vi "Main-Page.vi"() -> ()   [LabVIEW 2015]
uses:
  2.Queue/Control_Main_Queue Action.ctl
  <vilib>/Utility/miscctls.llb/LVPointTypeDef.ctl
  2.0_Function/Function_VISA/Control/Control_Axis Number.ctl
panel:
  out "data":T1(ring)
  in  "使用者帳戶":path=path "D:/全域高斯機 參數/use history"
  in  "參數設定":path=path "D:/全域高斯機 參數/use history"
  out "狀態：":string="可使用"
  out "群組：":string="開發人員"
  in  "原點資訊":path=path "D:/全域高斯機 參數/Original"
  in  "匯入硬體參數":path=path "D:/全域高斯機 參數/use history"
  in  "儲存檔案路徑":path=path "D:/全域高斯機Data"
  in  "匯入圖檔(Setting)":path=path "D:/全域高斯機資料/TAHOE3.png"
  out "狀態：":T2
  in  "離開程式":bool
  out "群組：":T3
  out "帳號：":string="admin"
  out "Queue Action":T4=enum."    10.2 系統-等待"
  in  "關於本系統":bool
  in  "資料管理":bool
  in  "登出/離開":bool
  in  "系統管理選單":bool
  in  "開始":bool
  in  "每日檢測":bool
  # "C:\\Users\\jyun.huang.MINAIK\\Desktop\\四穴雷切\\參數設定\\Data\\參數設定"
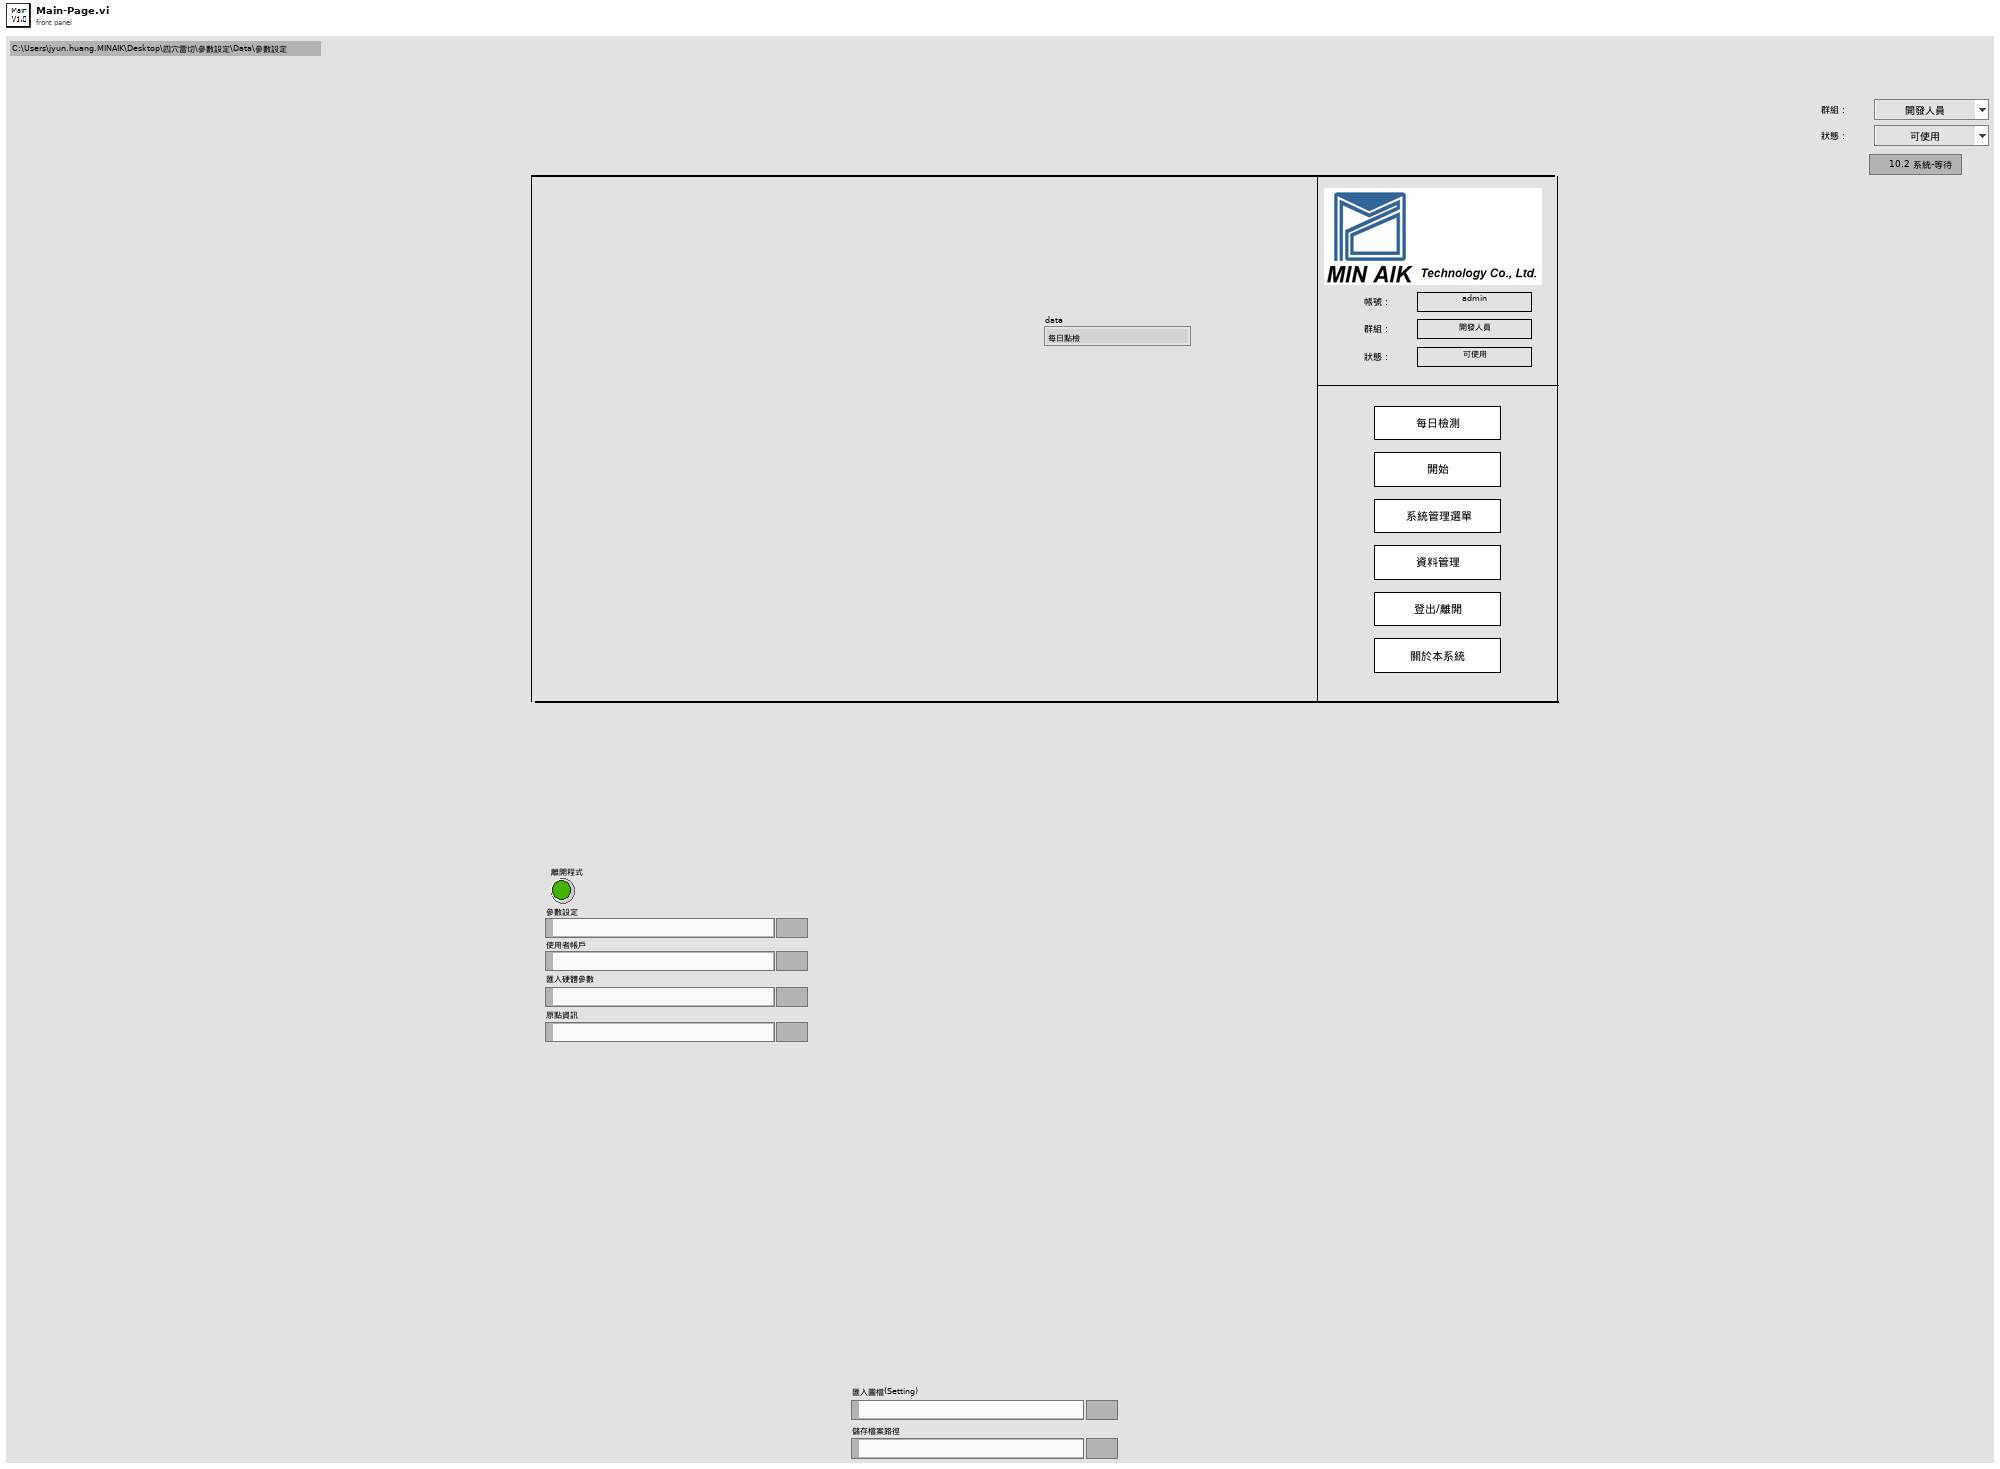
[diagram p1: front panel]
types:
  T1 = enum16{"每日點檢", "開始", "系統管理選單", "資料管理", "登出/離開", "關於本系統"}
  T2 = typedef "Control_User Accounts_Status.ctl" = enum16{"可使用", "不可使用"}
  T3 = typedef "Control_User account_Permissions.ctl" = enum16{"開發人員", "管理者", "工程師", "作業員"}
  T4 = typedef "Control_Main_Queue Action.ctl" = enum16{"動作-使用者登入", "動作-系統初始化", "動作-開始", "動作-系統管理選單", "動作-資料管理", "動作-登出/離開", "動作-關於本系統", "1.0 帳號管理", "    1.1 登入", "    1.2 確認狀態", "    1.3 更新介面", "    1.4 帳號管理", "    1.5 登出", "2.0 每日點檢", "10.0 系統", "    10.1 系統-關機", "    10.2 系統-等待", "    10.3 系統-回到作業系統"}
  T5 = cluster{string, "按鈕":enum16{"每日點檢", "開始", "系統管理選單", "資料管理", "登出/離開", "關於本系統"}}
  T6 = cluster{string, "系統":enum16{"關機", "等待", "回到作業系統"}}
  T7 = cluster{string, "帳號管理":enum16{"登入", "確認狀態", "更新介面", "帳號管理", "登出"}}
  T8 = typedef "LVPointTypeDef.ctl" = cluster{"Horizontal":i16, "Vertical":i16}
  T9 = typedef "Control_Original.ctl" = cluster{"R":dbl, "Y":dbl, "Z":dbl, "Angle":dbl}
  T10 = typedef "Control_軸參數.ctl" = cluster{"Name":string, "VISA In":refnum<visa-resource-name>, "R":dbl, "Y":dbl, "Z":dbl, "θ":dbl, "最大值":dbl, "最小值":dbl, "VISA Data":cluster{"Baud rate":u32, "Data bits":u16, "Parity":enum16{"None", "Odd", "Even", "Mark", "Space"}, "Stop bits":u16, "Flow control":u16}, "Paremeter":T11, "DAQ Paremeter":cluster{"Task In":refnum<k21>, "Physical Channels":tag, "Max Value":dbl, "Min Value":dbl, "Rate":dbl}}
  T11 = typedef "Control_手動測試_軸參數.ctl" = cluster{"Scan speed":T12, "Power":u16, "Angle":dbl, "X":i32, "X":i32, "Xc":i32}
  T12 = typedef "Control_Axis Number.ctl" = u16
  T13 = typedef "Control_Main_All Data.ctl" = enum16{"Initialize", "Set Data", "Get Data"}
  T14 = typedef "Use History.ctl" = enum16{"Initialize", "Set Data", "Get Data", "Idle"}
  T15 = typedef "Control_User account_Data.ctl" = cluster{"帳號 :":string, "權限等級：":T3, "建立時間：":string, "修改時間：":string, "到期時間：":string, "狀態：":T2, "期限：":T16, "密碼：":string}
  T16 = typedef "Control_User account_Date.ctl" = enum16{"零天", "一天", "七天", "一個月", "一年", "三年"}
  T17 = typedef "Action_Data.ctl" = enum16{"Initialize", "Get Data", "Set Data", "Delete Data", "Idle"}
  T18 = cluster{cluster{"掃描速度":i32, "功率":i32, "切割刀數":dbl, "左/右":string}, cluster{"掃描速度2":i32, "功率2":i32, "切割刀數2":dbl, "左/右":string}, cluster{"掃描速度3":i32, "功率3":i32, "切割刀數3":dbl, "左/右":string}, cluster{"掃描速度4":i32, "功率4":i32, "切割刀數4":dbl, "左/右":string}, cluster{"掃描速度5":i32, "功率5":i32, "切割刀數5":dbl, "左/右":string}}
  T19 = enum16{"All Enable", "All Disable", "Port Enable", "Port Disable"}
  T20 = typedef "Control_Bounce Window_Main_System Configuration.ctl" = enum16{"帳號管理", "手動操作", "機器參數設定", "離開", "等待"}
  T21 = typedef "Control_Bounce Window_Main_Data Management.ctl" = enum16{"量測參數設定", "操作履歷", "數據回顧", "離開", "等待"}
  T22 = typedef "Control_Bounce Window_Main_Log On-Exit.ctl" = enum16{"回到作業系統", "關機", "使用者登出", "離開", "等待"}
  T23 = cluster{"掃描速度5":i32, "功率5":i32, "切割刀數5":dbl, "左/右":string}
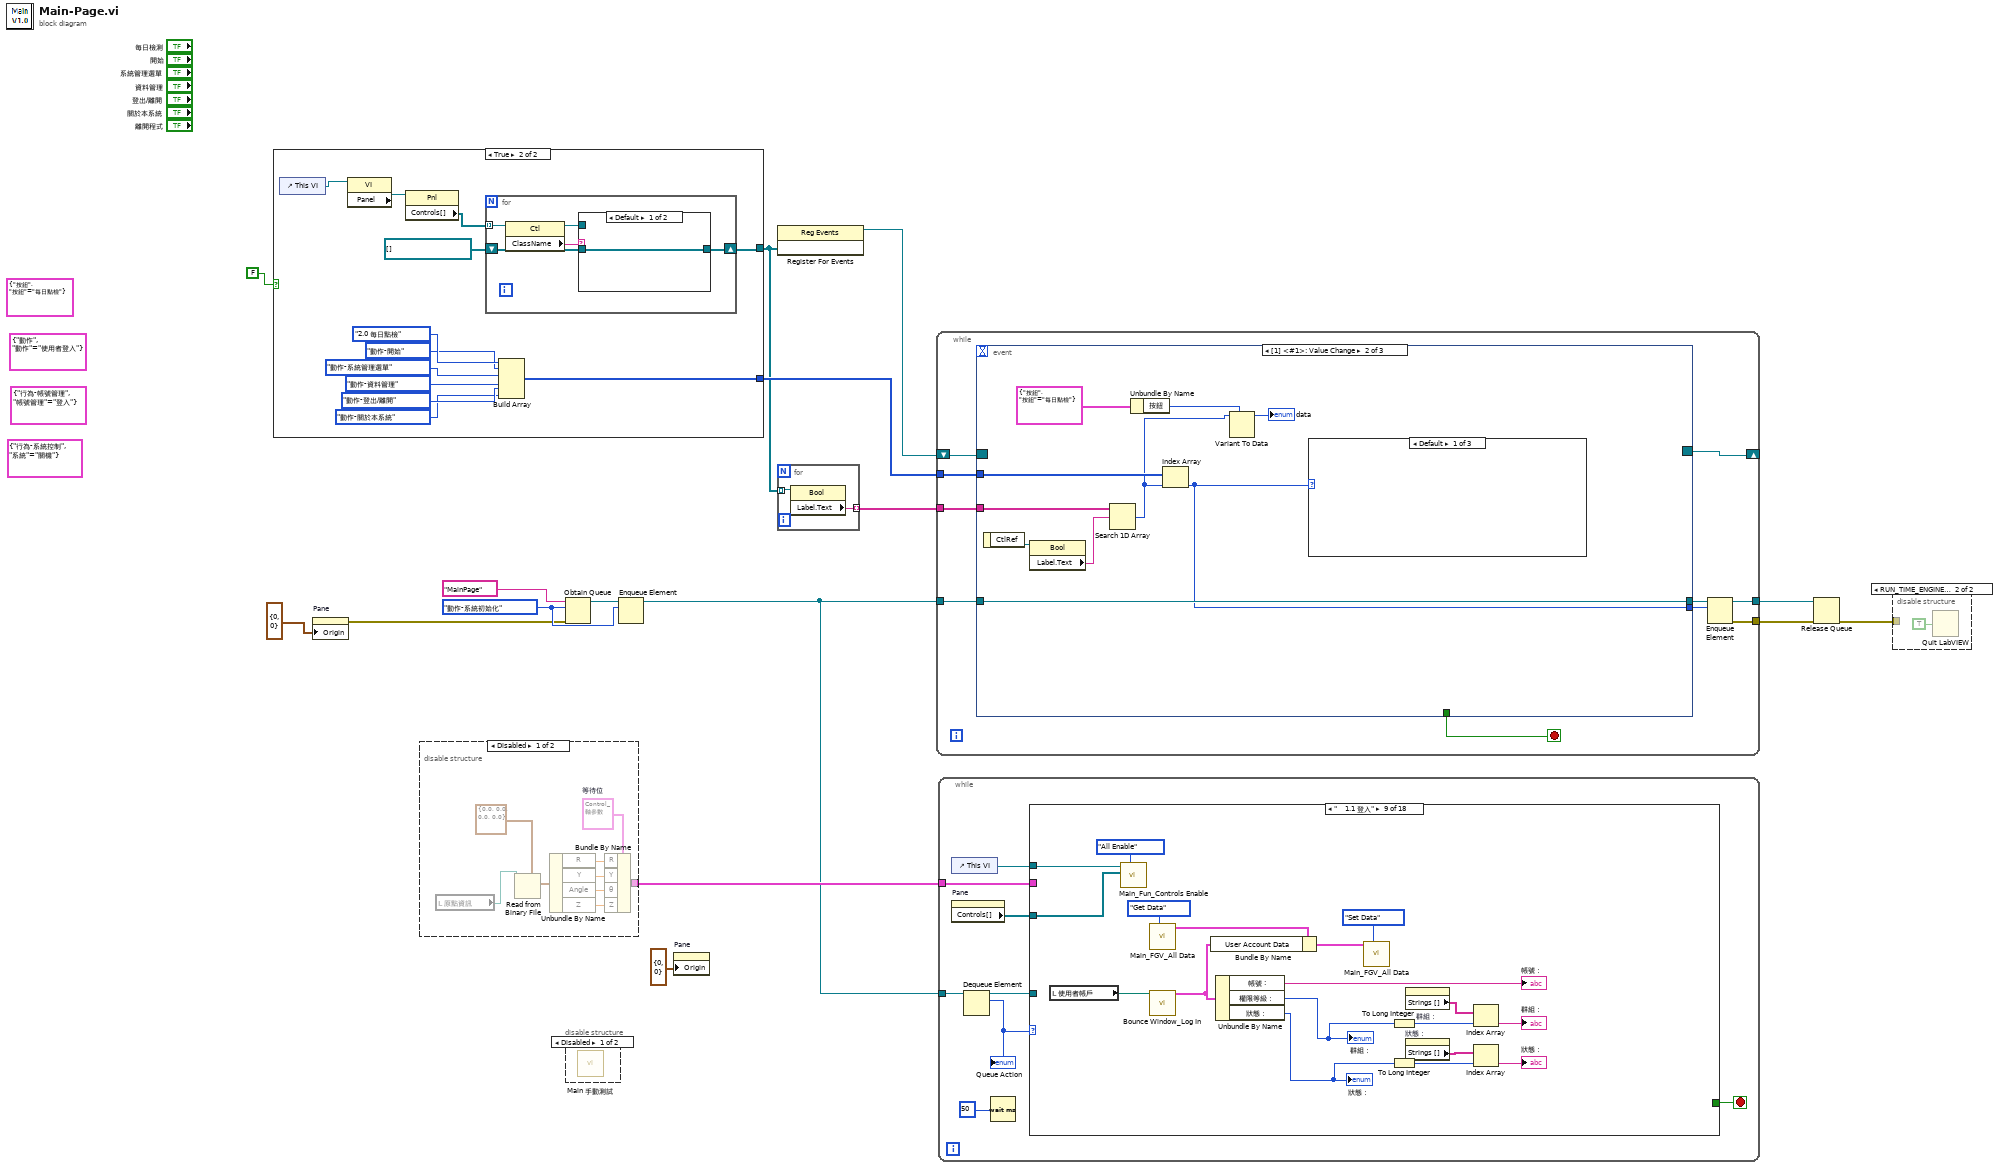
[diagram p0: block diagram]
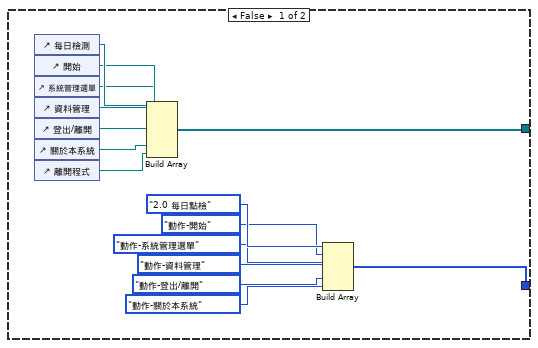
[diagram p2: hidden frame]
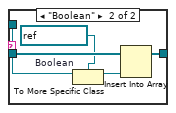
[diagram p3: hidden frame]
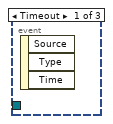
[diagram p4: hidden frame]
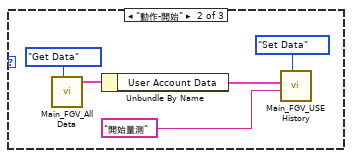
[diagram p5: hidden frame]
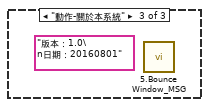
[diagram p6: hidden frame]
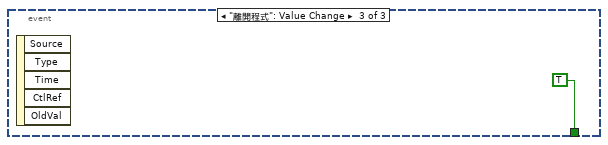
[diagram p7: hidden frame]
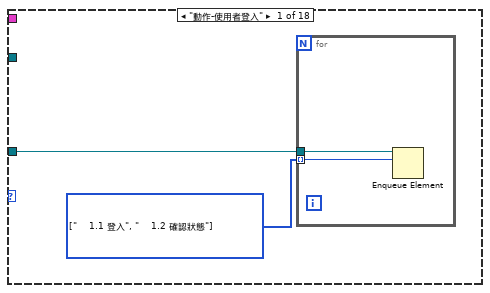
[diagram p11: hidden frame]
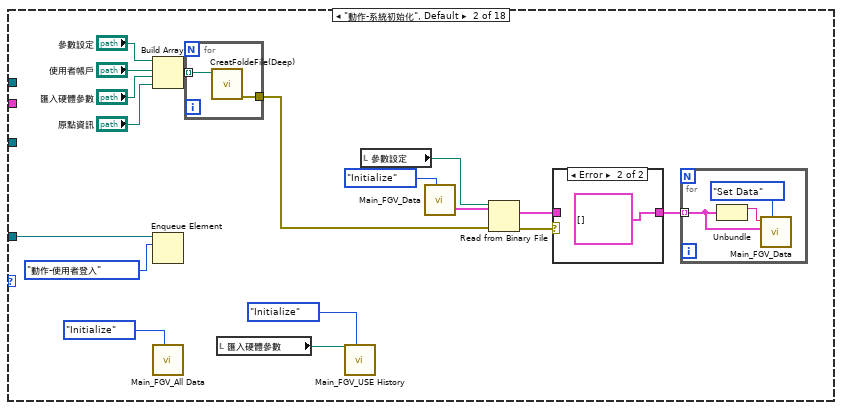
[diagram p12: hidden frame]
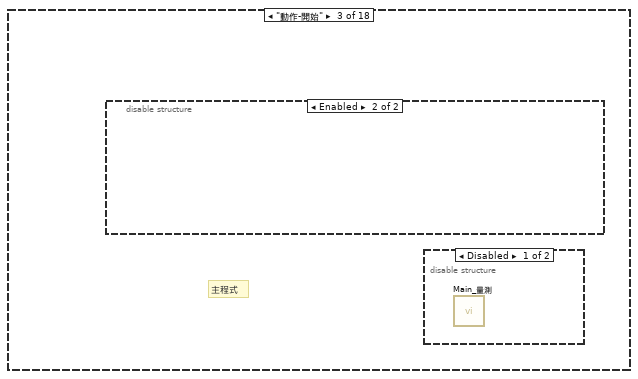
[diagram p14: hidden frame]
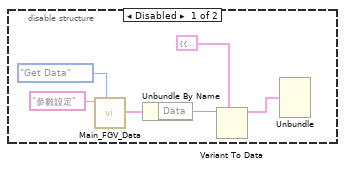
[diagram p16: hidden frame]
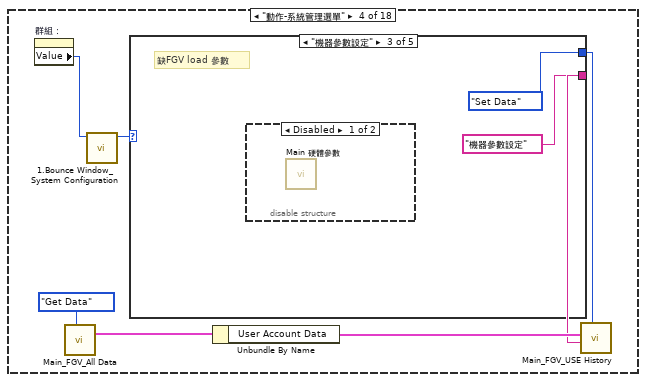
[diagram p17: hidden frame]
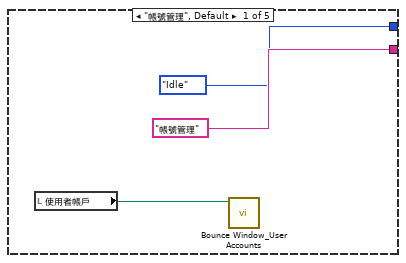
[diagram p18: hidden frame]
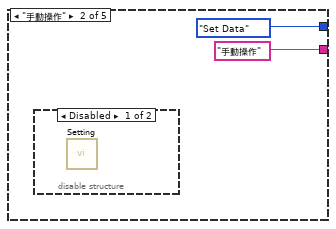
[diagram p19: hidden frame]
diagram:
  (unwired) T5 {"按鈕", "按鈕"=enum."每日點檢"} ("output cluster")
  (unwired) T6 {"行為-系統控制", "系統"=enum."關機"} ("output cluster")
  (unwired) T7 {"行為-帳號管理", "帳號管理"=enum."登入"} ("output cluster")
  (unwired) cluster{string, "動作":enum16{"使用者登入", "系統初始化"}} {"動作", "動作"=enum."使用者登入"} ("output cluster")
  w11 = Control_Main_Queue_Action."動作-系統初始化" ("Queue Action")
  n1 = case shown="True" FALSE {
    tunnel: [w17 w39] -> w3
    tunnel: [w18 w32] -> w6
    frame False {
      n2 = control-ref of="每日檢測"() -> (w31:refnum<vi>)
      n3 = control-ref of="開始"() -> (w30:refnum<vi>)
      n4 = control-ref of="系統管理選單"() -> (w29:refnum<vi>)
      n5 = control-ref of="資料管理"() -> (w28:refnum<vi>)
      n6 = control-ref of="登出/離開"() -> (w27:refnum<vi>)
      n7 = control-ref of="關於本系統"() -> (w26:refnum<vi>)
      n8 = control-ref of="離開程式"() -> (w25:refnum<vi>)
      n9 = Build Array(w31, w30, w29, w28, w27, w26, w25) -> (w17:refnum<vi>[])
      n10 = Build Array(Control_Main_Queue_Action."2.0 每日點檢" ("Queue Action"), Control_Main_Queue_Action."動作-開始" ("Queue Action"), Control_Main_Queue_Action."動作-系統管理選單" ("Queue Action"), Control_Main_Queue_Action."動作-資料管理" ("Queue Action"), Control_Main_Queue_Action."動作-登出/離開" ("Queue Action"), Control_Main_Queue_Action."動作-關於本系統" ("Queue Action")) -> (w18:T4[])
    }
    frame True {
      n11 = control-ref of="This VI"() -> (w43:refnum<vi>)
      n12 = property class="VI"(reference=w43) -> ("Panel"=w42:refnum<vi>)  [unwired: 1 in, 2 out]
      n13 = property class="Pnl"(reference=w42) -> ("Controls[]"=w41:refnum<vi>[])  [unwired: 1 in, 2 out]
      n14 = for {
        tunnel: w41 -> [w46] mode=indexing
        shift-right: [w45] -> w39
        shift-left: refnum<vi>[] [] -> [w47]
        n15 = property class="Ctl"(reference=w46) -> ("ClassName"=w44:string)  [unwired: 1 in, 2 out]
        n16 = case shown="Default" w44 {
          tunnel: w47 -> [w48 w53]
          tunnel: w46 -> [_ w52]
          tunnel: [w48 w50] -> w45
          frame Default {
          }
          frame "Boolean" {
            w51 = refnum<vi> refnum  # Boolean
            n17 = To More Specific Class(target class=w51, reference=w52) -> (specific class reference=w49:refnum<vi>)  [unwired: 1 in, 1 out]
            n18 = Insert Into Array(array=w53, new element=w49) -> (w50:refnum<vi>[])  [unwired: 1 in]
          }
        }
      }
      n19 = Build Array(Control_Main_Queue_Action."2.0 每日點檢" ("Queue Action"), Control_Main_Queue_Action."動作-開始" ("Queue Action"), Control_Main_Queue_Action."動作-系統管理選單" ("Queue Action"), Control_Main_Queue_Action."動作-資料管理" ("Queue Action"), Control_Main_Queue_Action."動作-登出/離開" ("Queue Action"), Control_Main_Queue_Action."動作-關於本系統" ("Queue Action")) -> (w32:T4[])
    }
  }
  n20 = property on="Pane" class="Pane"("Origin"=T8 {"Horizontal"=0, "Vertical"=0}) -> (error out=w10:errorcluster)  [unwired: 2 in, 1 out]
  n21 = disable-structure shown="Disabled" {
    disable-tunnel: [w55 _] -> w14
    frame Disabled {
      w56 = T10 {"Name"="", "VISA In"="COM2", "R"=40.8, "Y"=12.9, "Z"=0.0, "θ"=87.62, "最大值"=0.0, "最小值"=0.0, "VISA Data"={"Baud rate"=115200, "Data bits"=8, "Parity"=enum."Even", "Stop bits"=10, "Flow control"=0}, "Paremeter"={"Scan speed"=4, "Power"=2, "Angle"=0.0, "X"=9000, "X"=60000, "Xc"=60000}, "DAQ Paremeter"={"Task In"="CalibrationTest", "Physical Channels"="Dev1/ai0", "Max Value"=10.0, "Min Value"=-10.0, "Rate"=1000.0}}  # 等待位
      n22 = local read "原點資訊"() -> (w54:path)
      n23 = Read from Binary File(5:T9 {"R"=0.0, "Y"=0.0, "Z"=0.0, "Angle"=0.0} ("治具原點"), 11:w54) -> (2:w61:T9)  [unwired: 4 in, 3 out]
      n24 = Unbundle By Name(w61) -> ("R"=w60:dbl, "Y"=w59:dbl, "Angle"=w58:dbl, "Z"=w57:dbl)
      n25 = Bundle By Name(cluster=w56, "R"=w60, "Y"=w59, "θ"=w58, "Z"=w57) -> (w55:T10)
    }
    frame Enabled {
    }
  }
  n26 = Obtain Queue(name (unnamed)="MainPage", element data type=w11, error in (no error)=w10) -> (queue out=w12:refnum<queue>)  [unwired: 2 in, 2 out]
  n27 = disable-structure shown="Disabled" {
    frame Disabled {
      n28 = call "Main 手動測試.vi"() -> ()  [unwired: 12 in]
    }
    frame Enabled {
    }
  }
  n29 = Enqueue Element(queue=w12, element=w11) -> (queue out=w7:refnum<queue>)  [unwired: 2 in, 2 out]
  n30 = property on="Pane" class="Pane"("Origin"=T8 {"Horizontal"=0, "Vertical"=0}) -> ()  [unwired: 2 in, 2 out]
  n31 = register-events(w3) -> (reference out=w9:refnum<event-registration>)  [unwired: 2 in, 1 out]
  n32 = for {
    tunnel: w3 -> [w64] mode=indexing
    tunnel: [w63] -> w2 mode=indexing
    n33 = property class="Bool"(reference=w64) -> ("Label.Text"=w63:string)  [unwired: 1 in, 2 out]
  }
  n34 = while {
    shift-right: [w73] -> _
    shift-left: w9 -> [w74]
    tunnel: w2 -> [w72]
    tunnel: w7 -> [w70]
    tunnel: w6 -> [w68]
    tunnel: [w67] -> w5
    tunnel: [w66] -> w4
    stop <- w65 stop-if-true
    n35 = event shown="[1] <#1>: Value Change" {
      selector: w74 -> [_ _ _]
      dyn-events: [_ _ _] -> w73
      timeout: _ -> [_ _ _]
      tunnel: w72 -> [_ w84 _]
      tunnel: [_ w82 _] -> w71
      tunnel: w70 -> [_ w82 _]
      tunnel: [_ w76 _] -> w69
      tunnel: w68 -> [_ w81 _]
      tunnel: [_ _ TRUE] -> w65
      event Timeout {
        n36 = event-data() -> ()  [unwired: 1 in, 3 out]
      }
      event Value Change {
        n37 = event-data() -> ("CtlRef"=w80:refnum<vi>)  [unwired: 1 in]
        n38 = property class="Bool"(reference=w80) -> ("Label.Text"=w83:string)  [unwired: 1 in, 2 out]
        n39 = Search 1D Array(1D array=w84, element=w83) -> (index of element=w75:i32)  [unwired: 1 in]
        n40 = Unbundle By Name(T5 {"按鈕", "按鈕"=enum."每日點檢"} ("output cluster")) -> ("按鈕"=w78:T1)
        n41 = Index Array(array=w81, index=w75) -> (element=w76:T4)
        n42 = Variant To Data(type=w78, Variant=w75) -> (data=→"data":T1)  [unwired: 1 in, 1 out]
        n43 = case shown="Default" w76 {
          frame Default {
          }
          frame "動作-開始" {
            n44 = call "Main_FGV_All Data.vi"("Data_Action"=Control_Main_All_Data."Get Data") -> ("All Data Out"=w85:cluster{"User Account Data":T15})  [unwired: 9 in, 1 out]
            n45 = Unbundle By Name(w85) -> ("User Account Data"=w88:T15)
            n46 = call "Main_FGV_USE History.vi"("Use Action"=Use_History."Set Data", "Event"="開始量測", "User Account Data"=w88) -> ()  [unwired: 8 in, 1 out]
          }
          frame "動作-關於本系統" {
            (unwired) "版本：1.0\n日期：20160801" ("MSG In")
            n47 = call "5.Bounce Window_MSG.vi"() -> ()  [unwired: 12 in]
          }
        }
      }
      event "離開程式": Value Change {
        n48 = event-data() -> ()  [unwired: 1 in, 5 out]
      }
    }
    n49 = Enqueue Element(queue=w71, element=w69) -> (queue out=w67:refnum<queue>, error out=w66:errorcluster)  [unwired: 2 in, 1 out]
  }
  n50 = while {
    tunnel: w7 -> [w93]
    tunnel: w14 -> [w95]
    stop <- w98 stop-if-true
    n51 = control-ref of="This VI"() -> (w97:refnum<vi>)
    n52 = property on="Pane" class="Pane"() -> ("Controls[]"=w96:refnum<vi>[])  [unwired: 2 in, 2 out]
    n53 = Dequeue Element(queue=w93) -> (queue out=w92:refnum<queue>, element=w91:T4)  [unwired: 2 in, 2 out]
    "Queue Action" <- w91
    n54 = Wait (ms)(milliseconds to wait=u32 50) -> ()  [unwired: 1 out]
    n55 = case shown="\"    1.1 登入\"" w91 {
      tunnel: [_ _ _ _ _ _ _ _ _ _ _ _ _ _ TRUE _ TRUE _] -> w98
      tunnel: w92 -> [w100 w104 _ _ _ w166 _ _ _ w215 _ _ _ _ _ _ _ _]
      tunnel: w97 -> [_ _ _ _ _ _ _ _ w197 w209 _ _ _ _ _ _ _ _]
      tunnel: w96 -> [_ _ _ _ _ _ _ _ w196 w208 _ _ _ _ _ _ _ _]
      tunnel: w95 -> [_ _ _ _ w151 _ _ _ _ _ _ _ _ _ _ _ _ _]
      frame "動作-使用者登入" {
        w99 = T4[] [enum."    1.1 登入", enum."    1.2 確認狀態"] items=["動作-使用者登入", "動作-系統初始化", "動作-開始", "動作-系統管理選單", "動作-資料管理", "動作-登出/離開", "動作-關於本系統", "1.0 帳號管理", "    1.1 登入", "    1.2 確認狀態", "    1.3 更新介面", "    1.4 帳號管理", "    1.5 登出", "2.0 每日點檢", "10.0 系統", "    10.1 系統-關機", "    10.2 系統-等待", "    10.3 系統-回到作業系統"]
        n56 = for {
          tunnel: w100 -> [w102]
          tunnel: w99 -> [w101] mode=indexing
          n57 = Enqueue Element(queue=w102, element=w101) -> ()  [unwired: 2 in, 3 out]
        }
      }
      frame "動作-系統初始化", Default {
        n58 = Build Array("參數設定", "使用者帳戶", "匯入硬體參數", "原點資訊") -> (w119:path[])
        n59 = Enqueue Element(queue=w104, element=Control_Main_Queue_Action."動作-使用者登入" ("Queue Action")) -> ()  [unwired: 2 in, 3 out]
        n60 = call "Main_FGV_All Data.vi"("Data_Action"=Control_Main_All_Data."Initialize") -> ()  [unwired: 9 in, 2 out]
        n61 = for {
          tunnel: w119 -> [w126] mode=indexing
          tunnel: [w125] -> w110
          n62 = call "CreatFoldeFile(Deep).vi"("Path"=w126) -> ("error out"=w125:errorcluster)  [unwired: 8 in, 2 out]
        }
        n63 = local read "匯入硬體參數"() -> (w109:path)
        n64 = call "Main_FGV_USE History.vi"("Use Action"=Use_History."Initialize", "匯入硬體參數"=w109) -> ()  [unwired: 9 in, 1 out]
        n65 = local read "參數設定"() -> (w112:path)
        n66 = call "Main_FGV_Data.vi"("Action_Data"=Action_Data."Initialize") -> ("Data Array out"=w111:cluster{"Data name":string, "Data":variant}[])  [unwired: 9 in, 1 out]
        n67 = Read from Binary File(5:w111, 8:w110, 11:w112) -> (0:w107:errorcluster, 2:w106:cluster{"Data name":string, "Data":variant}[])  [unwired: 3 in, 2 out]
        n68 = case shown="Error" w107 {
          tunnel: w106 -> [w120 _]
          tunnel: [w120 cluster{"Data name":string, "Data":variant}[] [] ("Data Array out")] -> w105
          frame No Error {
          }
          frame Error {
          }
        }
        n69 = for {
          tunnel: w105 -> [w122] mode=indexing
          n70 = Unbundle(w122) -> ("Data name"=w123:string)  [unwired: 1 out]
          n71 = call "Main_FGV_Data.vi"("Action_Data"=Action_Data."Set Data", "Data In"=w122, "Data name"=w123) -> ()  [unwired: 7 in, 2 out]
        }
      }
      frame "動作-開始" {
        # "主程式"
        n72 = disable-structure shown="Enabled" {
          frame Disabled {
            n73 = call "Main_FGV_Data.vi"("Action_Data"=Action_Data."Get Data", "Data name"="參數設定") -> ("Data  Out"=w130:cluster{"Data name":string, "Data":variant})  [unwired: 8 in, 1 out]
            n74 = Unbundle By Name(w130) -> ("Data"=w129:variant)
            n75 = Variant To Data(type=T18 {{"掃描速度"=0, "功率"=0, "切割刀數"=0.0, "左/右"=""}, {"掃描速度2"=0, "功率2"=0, "切割刀數2"=0.0, "左/右"=""}, {"掃描速度3"=0, "功率3"=0, "切割刀數3"=0.0, "左/右"=""}, {"掃描速度4"=0, "功率4"=0, "切割刀數4"=0.0, "左/右"=""}, {"掃描速度5"=0, "功率5"=0, "切割刀數5"=0.0, "左/右"=""}} ("output cluster"), Variant=w129) -> (data=w128:T18)  [unwired: 1 in, 1 out]
            n76 = Unbundle(w128) -> ()  [unwired: 5 out]
          }
          frame Enabled {
          }
        }
        n77 = disable-structure shown="Disabled" {
          frame Disabled {
            n78 = call "Main_量測.vi"() -> ()  [unwired: 11 in]
          }
          frame Enabled {
          }
        }
      }
      frame "動作-系統管理選單" {
        n79 = property on="群組：" class="Enum (strict)"() -> ("Value"=w134:T3)  [unwired: 2 in, 2 out]
        n80 = call "Main_FGV_All Data.vi"("Data_Action"=Control_Main_All_Data."Get Data") -> ("All Data Out"=w139:cluster{"User Account Data":T15})  [unwired: 9 in, 1 out]
        n81 = call "1.Bounce Window_System Configuration.vi"("群組："=w134) -> ("系統管理選單"=w133:T20)  [unwired: 10 in]
        n82 = case shown="\"機器參數設定\"" w133 {
          tunnel: ["帳號管理" ("Event") "手動操作" ("Event") "機器參數設定" ("Event") "" ("Event") "" ("Event")] -> w136
          tunnel: [Use_History."Idle" ("Use Action") Use_History."Set Data" ("Use Action") Use_History."Set Data" ("Use Action") Use_History."Idle" ("Use Action") Use_History."Idle" ("Use Action")] -> w137
          frame "帳號管理", Default {
            n83 = local read "使用者帳戶"() -> (w140:path)
            n84 = call "Bounce Window_User Accounts.vi"("User Account Table Path"=w140) -> ()  [unwired: 11 in]
          }
          frame "手動操作" {
            n85 = disable-structure shown="Disabled" {
              frame Disabled {
                n86 = call "Setting.vi"() -> ()  [unwired: 11 in]
              }
              frame Enabled {
              }
            }
          }
          frame "機器參數設定" {
            # "缺FGV load 參數"
            n87 = disable-structure shown="Disabled" {
              frame Disabled {
                n88 = call "Main 硬體參數.vi"() -> ()  [unwired: 11 in]
              }
              frame Enabled {
              }
            }
          }
          frame "離開" {
          }
          frame "等待" {
          }
        }
        n89 = Unbundle By Name(w139) -> ("User Account Data"=w138:T15)
        n90 = call "Main_FGV_USE History.vi"("Use Action"=w137, "Event"=w136, "User Account Data"=w138) -> ()  [unwired: 8 in, 1 out]
      }
      frame "動作-資料管理" {
        n91 = property on="群組：" class="Enum (strict)"() -> ("Value"=w152:T3)  [unwired: 2 in, 2 out]
        n92 = call "2.Bounce Window_Data Management.vi"("群組："=w152) -> ("資料管理選單"=w153:T21)  [unwired: 10 in]
        n93 = case shown="\"離開\"" w153 {
          tunnel: w151 -> [_ _ _ _]
          tunnel: [Use_History."Set Data" ("Use Action") Use_History."Set Data" ("Use Action") Use_History."Idle" ("Use Action") Use_History."Idle" ("Use Action")] -> w157
          tunnel: ["量測參數設定" ("Event") "操作履歷" ("Event") _ _] -> w158
          frame "量測參數設定", Default {
          }
          frame "操作履歷" {
            n94 = call "使用者紀錄.vi"() -> ()  [unwired: 12 in]
          }
          frame "離開" {
          }
          frame "等待" {
          }
        }
        n95 = call "Main_FGV_All Data.vi"("Data_Action"=Control_Main_All_Data."Get Data") -> ("All Data Out"=w154:cluster{"User Account Data":T15})  [unwired: 9 in, 1 out]
        n96 = Unbundle By Name(w154) -> ("User Account Data"=w156:T15)
        n97 = call "Main_FGV_USE History.vi"("Use Action"=w157, "Event"=w158, "User Account Data"=w156) -> ()  [unwired: 8 in, 1 out]
      }
      frame "動作-登出/離開" {
        n98 = property on="群組：" class="Enum (strict)"() -> ("Value"=w168:T3)  [unwired: 2 in, 2 out]
        n99 = call "Main_FGV_All Data.vi"("Data_Action"=Control_Main_All_Data."Get Data") -> ("All Data Out"=w170:cluster{"User Account Data":T15})  [unwired: 9 in, 1 out]
        n100 = call "3.Bounce Window_Log On&Exit.vi"("群組："=w168) -> ("登出/離開"=w167:T22)  [unwired: 10 in]
        n101 = case shown="\"關機\"" w167 {
          tunnel: [Control_Main_Queue_Action."    10.3 系統-回到作業系統" ("Queue Action") Control_Main_Queue_Action."    10.1 系統-關機" ("Queue Action") Control_Main_Queue_Action."動作-使用者登入" ("Queue Action") Control_Main_Queue_Action."    10.2 系統-等待" ("Queue Action") Control_Main_Queue_Action."    10.2 系統-等待" ("Queue Action")] -> w165
          tunnel: w170 -> [_ _ _ _ _]
          tunnel: [Use_History."Set Data" ("Use Action") Use_History."Set Data" ("Use Action") Use_History."Set Data" ("Use Action") Use_History."Idle" ("Use Action") Use_History."Idle" ("Use Action")] -> w172
          tunnel: ["回到作業系統" "關機" "登出" _ _] -> w173
          frame "回到作業系統", Default {
          }
          frame "關機" {
          }
          frame "使用者登出" {
          }
          frame "離開" {
          }
          frame "等待" {
          }
        }
        n102 = Unbundle By Name(w170) -> ("User Account Data"=w171:T15)
        n103 = call "Main_FGV_USE History.vi"("Use Action"=w172, "Event"=w173, "User Account Data"=w171) -> ()  [unwired: 8 in, 1 out]
        n104 = Enqueue Element(queue=w166, element=w165) -> ()  [unwired: 2 in, 3 out]
      }
      frame "動作-關於本系統" {
      }
      frame "1.0 帳號管理" {
      }
      frame "    1.1 登入" {
        n105 = local read "使用者帳戶"() -> (w187:path)
        n106 = call "Main_Fun_Controls Enable.vi"("Controls Action"=T19."All Enable", "Controls In"=w196, "This VI Reference"=w197) -> ()  [unwired: 9 in]
        n107 = call "Main_FGV_All Data.vi"("Data_Action"=Control_Main_All_Data."Get Data") -> ("All Data Out"=w202:cluster{"User Account Data":T15})  [unwired: 9 in, 1 out]
        n108 = call "Bounce Window_Log In.vi"("User Account Table Path"=w187) -> ("User Account Data Out"=w199:T15)  [unwired: 9 in, 1 out]
        n109 = Bundle By Name(cluster=w202, "User Account Data"=w199) -> (w200:cluster{"User Account Data":T15})
        n110 = Unbundle By Name(w199) -> ("帳號 :"=→"帳號：":string, "權限等級："=w190:T3, "狀態："=w188:T2)
        "群組：" <- w190
        "狀態：" <- w188
        n111 = call "Main_FGV_All Data.vi"("Data_Action"=Control_Main_All_Data."Set Data", "All Data In"=w200) -> ()  [unwired: 8 in, 2 out]
        n112 = To Long Integer(number=w190) -> (32bit integer=w191:i32)
        n113 = To Long Integer(number=w188) -> (32bit integer=w189:i32)
        n114 = property on="群組：" class="Enum (strict)"() -> ("Strings []"=w193:string[])  [unwired: 2 in, 2 out]
        n115 = property on="狀態：" class="Enum (strict)"() -> ("Strings []"=w192:string[])  [unwired: 2 in, 2 out]
        n116 = Index Array(array=w193, index=w191) -> (element=→"群組：":string)
        n117 = Index Array(array=w192, index=w189) -> (element=→"狀態：":string)
      }
      frame "    1.2 確認狀態" {
        n118 = call "Main_FGV_All Data.vi"("Data_Action"=Control_Main_All_Data."Get Data") -> ("All Data Out"=w217:cluster{"User Account Data":T15})  [unwired: 9 in, 1 out]
        n119 = Unbundle By Name(w217) -> ("User Account Data.到期時間："=w214:string, "User Account Data.狀態："=w211:T2, "User Account Data.權限等級："=w210:T3, "User Account Data"=w207:T15)
        n120 = Format Date/Time String(time format string (%c)="%Y/%m/%d") -> (date/time string=w213:string)  [unwired: 2 in]
        n121 = Greater Or Equal?(x=w214, y=w213) -> (x >= y?=w212:bool)
        n122 = case shown="True" w212 {
          tunnel: w215 -> [w220 w227]
          tunnel: w211 -> [_ w228]
          tunnel: [w220 w226] -> w206
          tunnel: [Control_Main_Queue_Action."動作-使用者登入" ("Queue Action") w225] -> w205
          tunnel: w210 -> [_ w224]
          tunnel: w209 -> [_ w223]
          tunnel: w208 -> [_ w222]
          tunnel: w207 -> [_ w221]
          frame False {
          }
          frame True {
            n123 = case shown="\"可使用\", Default" w228 {
              tunnel: w227 -> [w238 w244]
              tunnel: [w238 w244] -> w226
              tunnel: [Control_Main_Queue_Action."    10.2 系統-等待" ("Queue Action") Control_Main_Queue_Action."動作-使用者登入" ("Queue Action")] -> w225
              tunnel: w224 -> [w236 _]
              tunnel: w223 -> [w234 _]
              tunnel: w222 -> [w233 _]
              tunnel: w221 -> [w230 _]
              frame "可使用", Default {
                n124 = case shown="\"工程師\"" w236 {
                  tunnel: [string[] [] ("Control Name Array In") string[] [] ("Control Name Array In") string[] ["系統管理選"] ("Control Name Array In") string[] ["系統管理選單", "資料管理"] ("Control Name Array In")] -> w232
                  frame "開發人員", Default {
                  }
                  frame "管理者" {
                  }
                  frame "工程師" {
                  }
                  frame "作業員" {
                  }
                }
                n125 = call "Main_Fun_Controls Enable.vi"("Controls Action"=T19."Port Disable", "Control Name Array In"=w232, "Controls In"=w233, "This VI Reference"=w234) -> ()  [unwired: 8 in]
                n126 = call "Main_FGV_USE History.vi"("Use Action"=Use_History."Set Data", "Event"="登入", "User Account Data"=w230) -> ()  [unwired: 8 in, 1 out]
              }
              frame "不可使用" {
              }
            }
          }
        }
        n127 = Enqueue Element(queue=w206, element=w205) -> ()  [unwired: 2 in, 3 out]
      }
      frame "    1.3 更新介面" {
      }
      frame "    1.4 帳號管理" {
      }
      frame "    1.5 登出" {
      }
      frame "10.0 系統" {
      }
      frame "    10.1 系統-關機" {
        n128 = call <vilib>:"System Exec.vi"("run minimized? (F)"=FALSE, "wait until completion? (T)"=TRUE, "command line"="shutdown -s -f -t 00") -> ()  [unwired: 5 in, 4 out]
      }
      frame "    10.2 系統-等待" {
      }
      frame "    10.3 系統-回到作業系統" {
        n129 = property on="離開程式" class="Bool (strict)"("Val(Sgnl)"=TRUE ("Value (Signaling)")) -> ()  [unwired: 2 in, 2 out]
      }
      frame "2.0 每日點檢" {
        n130 = disable-structure shown="Enabled" {
          disable-tunnel: [w251 _] -> _
          frame Disabled {
            n131 = call "Main_FGV_Data.vi"("Action_Data"=Action_Data."Get Data", "Data name"="參數設定") -> ("Data  Out"=w255:cluster{"Data name":string, "Data":variant})  [unwired: 8 in, 1 out]
            n132 = Unbundle By Name(w255) -> ("Data"=w254:variant)
            n133 = Variant To Data(type=T18 {{"掃描速度"=0, "功率"=0, "切割刀數"=0.0, "左/右"=""}, {"掃描速度2"=0, "功率2"=0, "切割刀數2"=0.0, "左/右"=""}, {"掃描速度3"=0, "功率3"=0, "切割刀數3"=0.0, "左/右"=""}, {"掃描速度4"=0, "功率4"=0, "切割刀數4"=0.0, "左/右"=""}, {"掃描速度5"=0, "功率5"=0, "切割刀數5"=0.0, "左/右"=""}} ("output cluster"), Variant=w254) -> (data=w253:T18)  [unwired: 1 in, 1 out]
            n134 = Unbundle(w253) -> (w251:T23)  [unwired: 4 out]
          }
          frame Enabled {
          }
        }
        n135 = disable-structure shown="Disabled" {
          frame Disabled {
            n136 = call "點檢.vi"() -> ()  [unwired: 12 in]
          }
          frame Enabled {
          }
        }
      }
    }
  }
  n137 = Release Queue(queue=w5, error in (no error)=w4) -> (error out=w1:errorcluster)  [unwired: 1 in, 2 out]
  n138 = disable-structure shown="RUN_TIME_ENGINE==True" {
    disable-tunnel: w1 -> [_ _]
    frame condition #0 (active) {
    }
    frame condition #1 {
      n139 = Quit LabVIEW(quit? (T)=TRUE) -> ()
    }
  }
